vi "readPlungerStatus.vi"() -> (1 "plunger status":enum16{"ASSERTED", "DE-ASSERTED\nOUT OF BEAM"}[](array[ring]), 2 "read switches":T2[](array[typedef]), 3 "timed out":bool)   [LabVIEW 2020]
uses:
  plungerstatus.ctl
panel:
  out "time":u32
  out "DSRead_Error 1":errorcluster
  out "Status":T1={"bits 2"=[FALSE, FALSE, FALSE, FALSE, FALSE, FALSE, FALSE, FALSE, FALSE, FALSE, FALSE, FALSE, FALSE, FALSE, FALSE, FALSE, FALSE, FALSE, FALSE, FALSE, FALSE, FALSE, FALSE, FALSE, FALSE, FALSE, FALSE, FALSE, FALSE, FALSE, FALSE, FALSE, FALSE, FALSE, FALSE, FALSE, FALSE, FALSE, FALSE, FALSE, FALSE, FALSE, FALSE, FALSE, FALSE, FALSE, FALSE, FALSE, FALSE, FALSE, FALSE, FALSE, FALSE, FALSE, FALSE, FALSE, FALSE, FALSE, FALSE, FALSE, FALSE, FALSE, FALSE, FALSE], "bits 2"=[FALSE, FALSE, FALSE, FALSE, FALSE, FALSE, FALSE, FALSE, FALSE, FALSE, FALSE, FALSE, FALSE, FALSE, FALSE, FALSE, FALSE, FALSE, FALSE, FALSE, FALSE, FALSE, FALSE, FALSE, FALSE, FALSE, FALSE, FALSE, FALSE, FALSE, FALSE, FALSE], "bits 2"=[TRUE, FALSE, FALSE, FALSE, FALSE, FALSE, FALSE, FALSE, FALSE, FALSE, FALSE, FALSE, FALSE, FALSE, FALSE, FALSE], [0, 0, 0, 0, 0, 0]}
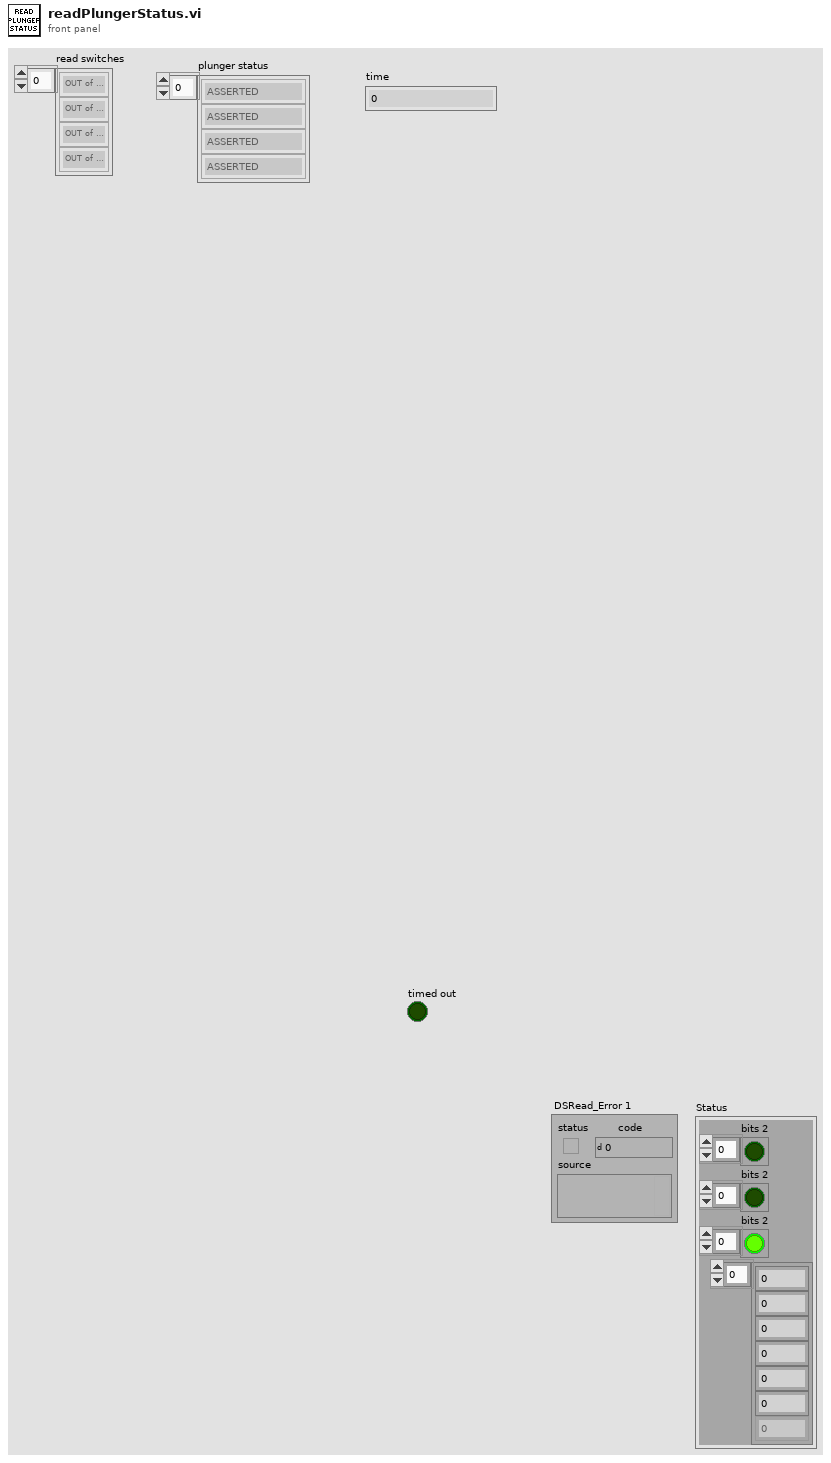
[diagram p1: front panel]
types:
  T1 = cluster{"bits 2":bool[], "bits 2":bool[], "bits 2":bool[], i32[]}
  T2 = typedef "plungerstatus.ctl" = enum16{"unknown", "OUT of Beam", "IN Beam"}
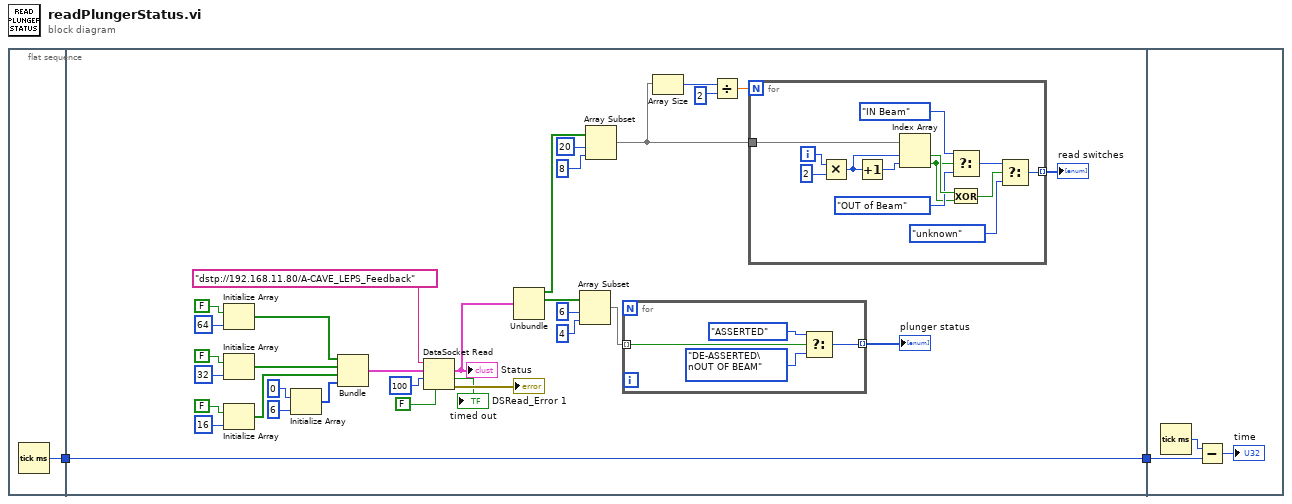
[diagram p0: block diagram]
diagram:
  n1 = flat-sequence {
    tunnel: [w3] -> w2
    tunnel: w2 -> [w18]
    tunnel: [w18] -> w1
    tunnel: w1 -> [w55]
    frame #0 {
      n2 = Tick Count (ms)() -> (millisecond timer value=w3:u32)
    }
    frame #1 {
      n3 = Initialize Array(FALSE, 64 ("size(s) 5")) -> (w10:bool[])
      n4 = Initialize Array(FALSE, 32 ("size(s) 5")) -> (w9:bool[])
      n5 = Initialize Array(FALSE, 16 ("size(s) 5")) -> (w8:bool[])
      n6 = Initialize Array(0, 6 ("size(s) 5")) -> (w5:i32[])
      n7 = Bundle(w10, w9, w8, w5) -> (w6:cluster{bool[], bool[], bool[], i32[]})  [unwired: 1 in]
      n8 = DataSocket Read(6:FALSE ("wait for updated value (T)"), 9:100 ("ms timeout (10000)"), 10:w6, 11:"dstp://192.168.11.80/A-CAVE_LEPS_Feedback" ("Source_URL")) -> (0:→"DSRead_Error 1":errorcluster, 1:→"timed out":bool, 2:w19:cluster{bool[], bool[], bool[], i32[]})  [unwired: 1 in, 4 out]
      "Status" <- w19
      n9 = Unbundle(w19) -> (w36:bool[], w25:bool[])  [unwired: 2 out]
      n10 = Array Subset(array=w25, index=6, length=4) -> (w24:bool[])
      n11 = Array Subset(array=w36, index=20, length=8) -> (w34:bool[])
      n12 = for {
        tunnel: [w38] -> w26 mode=indexing
        tunnel: w24 -> [w37] mode=indexing
        n13 = Select(t=enum16{"ASSERTED", "DE-ASSERTED\nOUT OF BEAM"}."ASSERTED", s=w37, f=enum16{"ASSERTED", "DE-ASSERTED\nOUT OF BEAM"}."DE-ASSERTED\nOUT OF BEAM") -> (s? t:f=w38:enum16{"ASSERTED", "DE-ASSERTED\nOUT OF BEAM"})
      }
      "plunger status" <- w26
      n14 = Array Size(array=w34) -> (size(s)=w31:i32)
      n15 = Divide(x=w31, y=2) -> (x/y=w29:dbl)
      n16 = for {
        N: w29 -> [_]
        tunnel: w34 -> [w53]
        tunnel: [w44] -> w33 mode=indexing
        i -> [w50]
        n17 = Multiply(x=w50, y=2) -> (x*y=w48:i32)
        n18 = Increment(x=w48) -> (x+1=w52:i32)
        n19 = Index Array(array=w53, index #1=w48, index #2=w52) -> (element #1=w47:bool, element #2=w45:bool)
        n20 = Select(t=plungerstatus."IN Beam", s=w45, f=plungerstatus."OUT of Beam") -> (s? t:f=w42:T2)
        n21 = Exclusive Or(1:w45, 2:w47) -> (0:w41:bool)
        n22 = Select(t=w42, s=w41, f=plungerstatus."unknown") -> (s? t:f=w44:T2)
      }
      "read switches" <- w33
    }
    frame #2 {
      n23 = Tick Count (ms)() -> (millisecond timer value=w56:u32)
      n24 = Subtract(x=w56, y=w55) -> (x-y=→"time":u32)
    }
  }
